vi "DSP Processing.vi"(8 "error in (no error)":errorcluster) -> (0 "error out":errorcluster)   [LabVIEW 2016]
uses:
  Utilities/Application Globals.vi
  <vilib>/Analysis/3filter.llb/Filter Passband Type.ctl
  <vilib>/Analysis/NI_AALBase.lvlib
  RTLSDR Control/RTLSDR Global Variables.vi
  <vilib>/ptbypt/NI_PtbyPt.lvlib
  FPGA Control/FPGA Global Variables.vi
  <vilib>/rvi/interface/nirviMethod/nirviMethod.xnode
  <vilib>/Analysis/3filter.llb/Butterworth Filter (CDB).vi
  <vilib>/FPGAPlugInAG/Dynamic/niLvFpga_WriteFifo_Dynamic.vi
  <vilib>/rvi/errors/niLvFpgaMergeErrorWithErrorCode.vi
panel:
  out "min value":dbl
  out "max value":dbl
  out "Empty Elements Remaining":u32
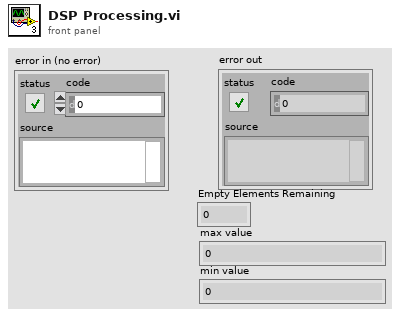
[diagram p1: front panel]
types:
  T1 = typedef "NI_AALBase.lvlib/Filter Passband Type.ctl" = enum32{"Lowpass", "Highpass", "Bandpass", "Bandstop"}
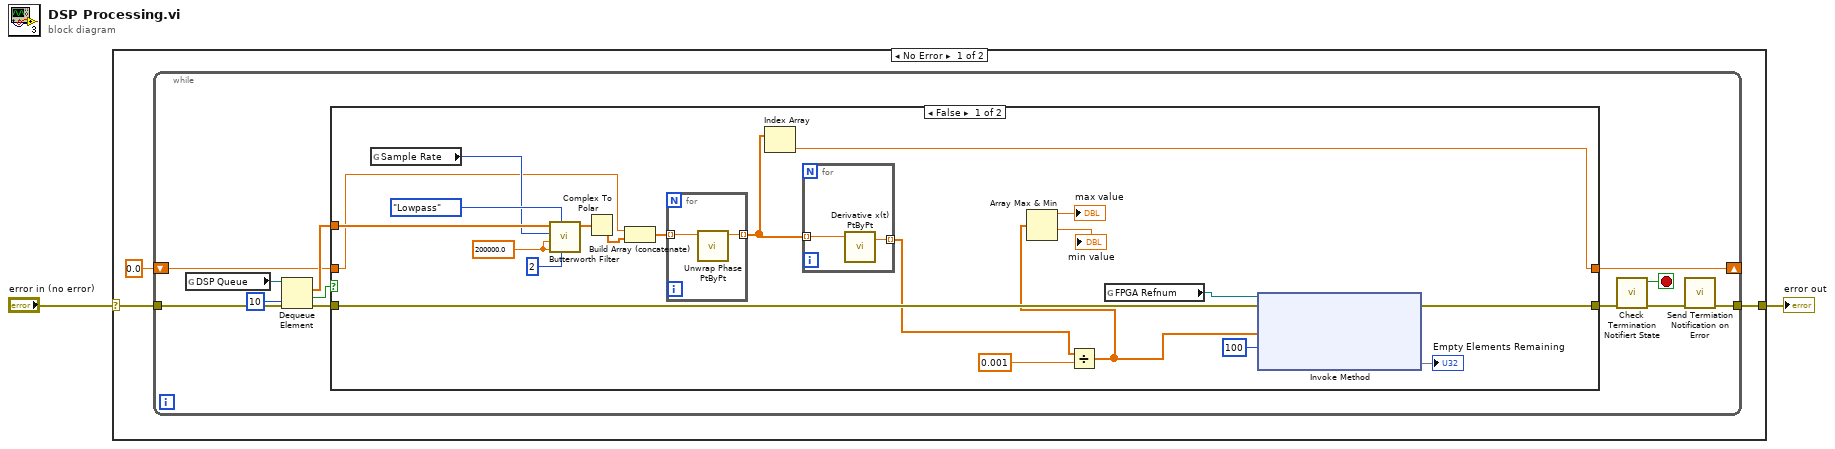
[diagram p0: block diagram]
diagram:
  n1 = case shown="No Error" "error in (no error)" {
    selector: "error in (no error)" -> [w5 w45]
    tunnel: [w4 w45] -> w1
    frame No Error {
      n2 = while {
        shift-right: [w14] -> _
        shift-left: 0.0 ("unwrapped phase") -> [w13]
        tunnel: w5 -> [w12]
        tunnel: [w9] -> w4
        stop <- w11 stop-if-true
        n3 = global read "Application Globals.vi" "DSP Queue"() -> (w17:refnum<queue>)
        n4 = Dequeue Element(queue=w17, timeout in ms (-1)=10, error in (no error)=w12) -> (element=w16:cdb[], timed out?=w15:bool, error out=w8:errorcluster)  [unwired: 1 out]
        n5 = case shown="False" w15 {
          tunnel: w16 -> [w38 _]
          tunnel: [w27 w44] -> w14
          tunnel: w13 -> [w25 w44]
          tunnel: w8 -> [w23 w43]
          tunnel: [w31 w43] -> w7
          frame False {
            w26 = 200000.0 ("low cutoff freq: fl")
            n6 = global read "RTLSDR Global Variables.vi" "Sample Rate"() -> (w33:u32)
            n7 = call-poly <vilib>:"Butterworth Filter.vi"("order"=2, "filter type"=Filter_Passband_Type."Lowpass", "low cutoff freq: fl"=w26, "high cutoff freq: fh"=w26, "sampling freq: fs"=w33, "X"=w38) -> ("Filtered X"=w36:cdb[])  [unwired: 2 in, 1 out]
            n8 = Complex To Polar(r * e^(i*theta)=w36) -> (theta=w24:dbl[])  [unwired: 1 out]
            n9 = Build Array (concatenate)(w25, w24) -> (w34:dbl[])
            n10 = for {
              tunnel: w34 -> [w42] mode=indexing
              tunnel: [w41] -> w28 mode=indexing
              n11 = call <vilib>:"Unwrap Phase PtByPt.vi"("phase"=w42) -> ("unwrapped phase"=w41:dbl)  [unwired: 10 in]
            }
            n12 = Index Array(array=w28) -> (element=w27:dbl)  [unwired: 1 in]
            n13 = for {
              tunnel: w28 -> [w40] mode=indexing
              tunnel: [w39] -> w20 mode=indexing
              n14 = call <vilib>:"Derivative x(t) PtByPt.vi"("x"=w40) -> ("dx/dt"=w39:dbl)  [unwired: 3 in, 1 out]
            }
            n15 = Divide(x=w20, y=0.001) -> (x/y=w18:dbl[])
            n16 = Array Max & Min(array=w18) -> (max value=→"max value":dbl, min value=→"min value":dbl)  [unwired: 2 out]
            n17 = global read "FPGA Global Variables.vi" "FPGA Refnum"() -> (w32:refnum<k20>)
            n18 = xnode "Invoke Method"("FPGA VI Reference In"=w32, "error in"=w23, "Data"=w18, "Timeout (ms)"=100) -> ("error out"=w31:errorcluster, "Empty Elements Remaining"=→"Empty Elements Remaining")  [unwired: 1 out]
          }
          frame True {
          }
        }
        n19 = call "Check Termination Notifiert State.vi"("error in (no error)"=w7) -> ("error out"=w10:errorcluster, "Termination Notifier State"=w11:bool)  [unwired: 9 in]
        n20 = call "Send Termiation Notification on Error.vi"("error in (no error)"=w10) -> ("error out"=w9:errorcluster)  [unwired: 10 in]
      }
    }
    frame Error {
    }
  }
  "error out" <- w1
